vi "PicoScope4000aExampleRapidBlockBulk.vi"() -> ()   [LabVIEW 2016]
uses:
  PicoScope4000aLib/PicoScope4000aAnalogChannelSettings.ctl
panel:
  out "USB 3.0 on non-USB 3.0 port":bool=TRUE
  out "USB powered":bool=TRUE
  in  "Trigger Settings":T1={"Trigger Enabled"=FALSE, "Trigger Source"=enum."Channel A", "Trigger Threshold (Volts/Probe Units)"=0.0, "Trigger Direction"=2, "Trigger Delay (samples)"=0, "Auto Trigger Time (ms)"=0} {"Trigger Direction" items=["Rising"=2, "Falling"=3]}
  in  "Resolution":u16(ring)=1 items=["12-bit"=1, "14-bit"=2]
  in  "Serial Number":string
  in  "Use Serial Number":bool
  out "Number of Samples \nPer Capture":u32
  in  "Channel A Settings":T2={"Enabled"=TRUE, "Coupling"=1, "Range"=6, "Analogue Offset"=0.0, "Bandwidth Limit"=0} {"Bandwidth Limit" items=["Full", "20kHz", "100kHz", "1MHz"]; "Range" items=["10 mV", "20 mV", "50 mV", "100 mV", "200 mV", "500 mV", "1 V", "2 V", "5 V", "10 V", "20 V", "50 V ", "100 V"]; "Coupling" items=["AC", "DC"]}
  in  "Rapid Block Acquisition Settings":T3={"preTriggerSamples"=512, "postTriggerSamples"=512, "timebase"=10, "Number of Captures"=64}
  out "Capture Complete":bool
  in  "Run":bool
  out "Channel A":i16[](graph)
  in  "Capture Index":i16 min=0
  in  "stop":bool
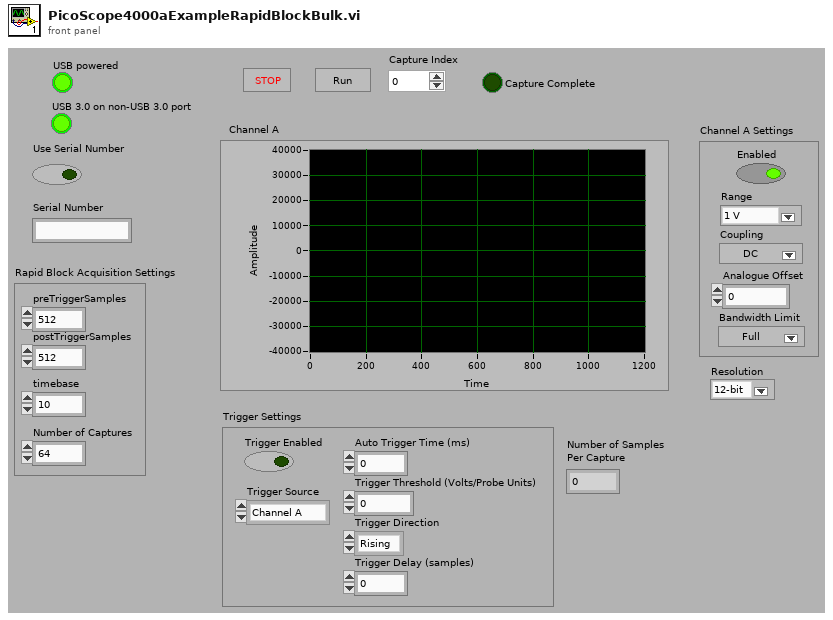
[diagram p1: front panel]
types:
  T1 = cluster{"Trigger Enabled":bool, "Trigger Source":enum16{"Channel A", "Channel B", "Channel C", "Channel D", "Channel E", "Channel F", "Channel G", "Channel H"}, "Trigger Threshold (Volts/Probe Units)":dbl, "Trigger Direction":u16, "Trigger Delay (samples)":u32, "Auto Trigger Time (ms)":i16}
  T2 = typedef "PicoScope4000aAnalogChannelSettings.ctl" = cluster{"Enabled":bool, "Coupling":i16, "Range":u16, "Analogue Offset":sgl, "Bandwidth Limit":u32}
  T3 = cluster{"preTriggerSamples":u32, "postTriggerSamples":u32, "timebase":u32, "Number of Captures":u32}
  T4 = cluster{"Driver Version":string, "USB Version":string, "Hardware":string, "Variant":string, "Batch and Serial":string, "Cal Date":string, "Kernel Version":string, "Digital HW Version":string, "Analogue HW Version":string, "Firmware 1":string, "Firmware 2":string, "Num. channels":i16}
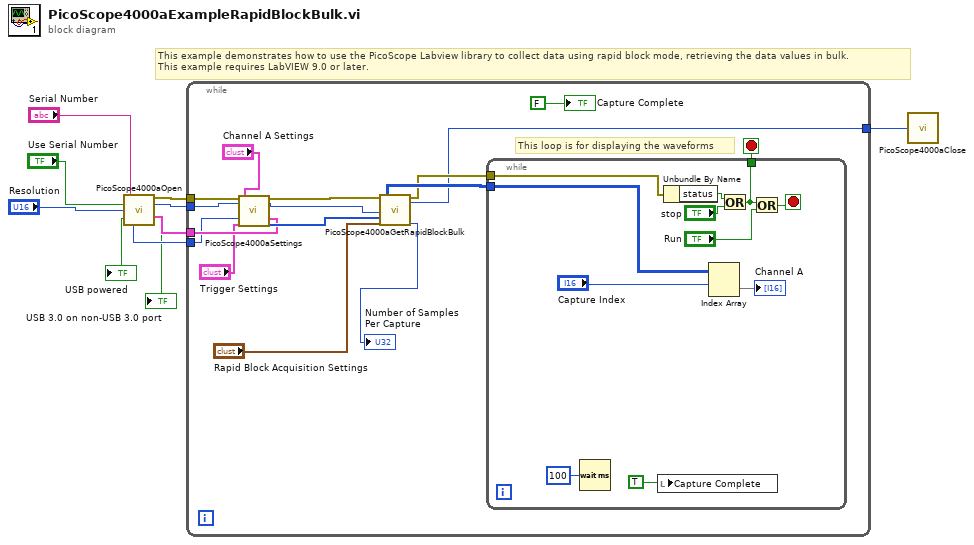
[diagram p0: block diagram]
diagram:
  # "This example demonstrates how to use the PicoScope Labview library to collect data using rapid block mode, retrieving the data values in bulk.\nThis example requires LabVIEW 9.0 or later."
  n1 = call "PicoScope4000aOpen.vi"("Serial Number"="Serial Number", "Use Serial Number"="Use Serial Number", "Resolution"="Resolution") -> ("error out"=w7:errorcluster, "handle"=w6:i16, "Unit Info"=w5:T4, "Max ADC value"=w3:i16, "USB powered"=→"USB powered":bool, "USB 3.0 on non-USB 3.0 port"=→"USB 3.0 on non-USB 3.0 port":bool)  [unwired: 7 in]
  n2 = while {
    tunnel: [w19] -> w10
    tunnel: w7 -> [w24]
    tunnel: w6 -> [w22]
    tunnel: w5 -> [w13]
    tunnel: w3 -> [w12]
    stop <- w26 stop-if-true
    # "This loop is for displaying the waveforms"
    n3 = call "PicoScope4000aSettings.vi"("error in"=w24, "handle in"=w22, "Max ADC value"=w12, "Trigger Settings"="Trigger Settings", "Channel A Settings"="Channel A Settings", "Unit Info"=w13) -> ("error out"=w17:errorcluster, "handle out"=w16:i16, "Enabled array"=w14:i16[])  [unwired: 11 in]
    n4 = call "PicoScope4000aGetRapidBlockBulk.vi"("error in"=w17, "handle in"=w16, "Enabled array"=w14, "Rapid Block Acquisition Settings"="Rapid Block Acquisition Settings") -> ("Channel A Buffer"=w21:i16[][], "error out"=w20:errorcluster, "handle out"=w19:i16, "Num samples"=→"Number of Samples \nPer Capture":u32)  [unwired: 4 in, 8 out]
    n5 = while {
      tunnel: [w36] -> w26
      tunnel: w21 -> [w29]
      tunnel: w20 -> [w31]
      stop <- w35 stop-if-true
      n6 = Wait (ms)(milliseconds to wait=u32 100) -> ()  [unwired: 1 out]
      n7 = local write "Capture Complete"(TRUE ("Capture Complete")) -> ()
      n8 = Unbundle By Name(w31) -> ("status"=w30:bool)
      n9 = Index Array(array=w29, index (row)="Capture Index") -> (element=→"Channel A":i16[])  [unwired: 1 in]
      n10 = Or(x=w30, y="stop") -> (x .or. y?=w36:bool)
      n11 = Or(x=w36, y="Run") -> (x .or. y?=w35:bool)
    }
    "Capture Complete" <- FALSE ("Capture Complete")
  }
  n12 = call "PicoScope4000aClose.vi"("handle"=w10) -> ()
